vi "List.vi"(8 "error in (no error)":errorcluster) -> (0 "error out":errorcluster, 3 "Modules":T1[](array[typedef]))   [LabVIEW 2018, in "Core.lvlib" / "Module.lvlib"]
uses:
  Module.lvlib
  Controls/Module.ctl
  Controls/Instance.ctl
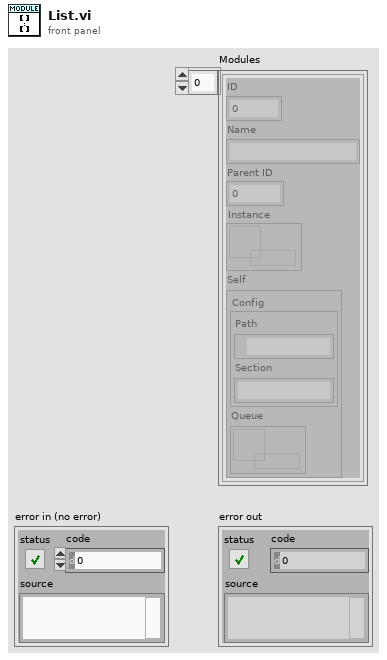
[diagram p1: front panel]
types:
  T1 = typedef "Core.lvlib/Module.lvlib/Module.ctl" = cluster{"ID":i32, "Name":string, "Parent ID":i32, "Instance":refnum<data-value>, "Self":T2}
  T2 = typedef "Core.lvlib/Module.lvlib/Instance.ctl" = cluster{"Config":cluster{"Path":path, "Section":string}, "Queue":refnum<queue>}
  T3 = cluster{"ID":i32, "Name":string, "Parent ID":i32, "Instance":refnum<data-value>}[]
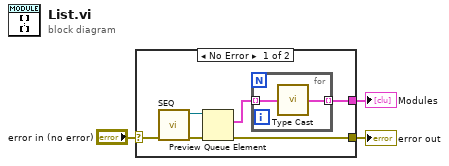
[diagram p0: block diagram]
diagram:
  n1 = case shown="No Error" "error in (no error)" {
    selector: "error in (no error)" -> [w9 w12]
    tunnel: [w4 w12] -> w2
    tunnel: [w6 _] -> w1
    frame No Error {
      n2 = call "SEQ.vi"("error in (no error)"=w9) -> ("error out"=w8:errorcluster, "Modules"=w7:refnum<queue>)  [unwired: 8 in, 1 out]
      n3 = Preview Queue Element(queue=w7, error in (no error)=w8) -> (element=w5:T3, error out=w4:errorcluster)  [unwired: 1 in, 2 out]
      n4 = for {
        tunnel: [w11] -> w6 mode=indexing
        tunnel: w5 -> [w10] mode=indexing
        n5 = call "Type Cast.vi"("Module in"=w10) -> ("Module"=w11:T1)
      }
    }
    frame Error {
    }
  }
  "error out" <- w2
  "Modules" <- w1
